vi "RSZVB Get Physical Port Trigger Delay.vi"(8 "error in (no error)":errorcluster {"code" format="%.0x"}, 9 "Analyzer Port (1)":i32=1, 10 "Channel (1)":i32=1, 11 "VISA session":refnum<visa-resource-name>) -> (0 "error out":errorcluster {"code" format="%.0x"}, 2 "Trigger Delay":dbl format="%^.3e", 3 "dup VISA session":refnum<visa-resource-name>)   [LabVIEW 2011]
doc: "Queries the trigger delay for a physical analyzer port <Pt>.\n\nRemote-control command(s):\nTRIGger<Ch>[:SEQuence]:HOLDoff:PORT<Pt>?"
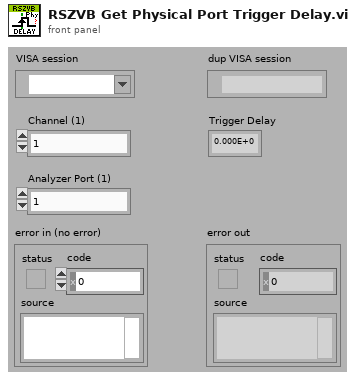
[diagram p1: front panel]
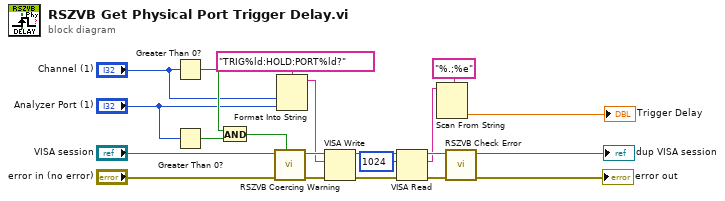
[diagram p0: block diagram]
diagram:
  n1 = Greater Than 0?(x="Channel (1)") -> (x > 0?=w16:bool)
  n2 = Greater Than 0?(x="Analyzer Port (1)") -> (x > 0?=w17:bool)
  n3 = And(x=w16, y=w17) -> (x .and. y?=w15:bool)
  n4 = call "RSZVB Coercing Warning.vi"("In Range?"=w15, "error in (no error)"="error in (no error)", "VISA session"="VISA session") -> ("error out"=w19:errorcluster, "dup VISA session"=w20:refnum<visa-resource-name>)  [unwired: 7 in]
  n5 = Format Into String(format string="TRIG%ld:HOLD:PORT%ld?", "Channel (1)", "Analyzer Port (1)") -> (resulting string=w18:string)  [unwired: 2 in, 1 out]
  n6 = VISA Write(VISA resource name=w20, write buffer=w18, error in (no error)=w19) -> (VISA resource name out=w13:refnum<visa-resource-name>, error out=w14:errorcluster)  [unwired: 1 out]
  n7 = VISA Read(VISA resource name=w13, byte count=u32 1024, error in (no error)=w14) -> (VISA resource name out=w11:refnum<visa-resource-name>, read buffer=w8:string, error out=w12:errorcluster)  [unwired: 1 out]
  n8 = Scan From String(format string="%.;%e", input string=w8) -> (output 1=→"Trigger Delay":dbl)  [unwired: 3 in, 3 out]
  n9 = call "RSZVB Check Error.vi"("error in (no error)"=w12, "VISA session"=w11) -> ("error out"=→"error out":errorcluster, "dup VISA session"=→"dup VISA session":refnum<visa-resource-name>)  [unwired: 8 in]
